vi "ref_gen.vi"(3 "xk":T1, 4 "error in (no error)":errorcluster, 5 "wd":dbl, 6 "B":T1, 7 "A":T1) -> (0 "error out":errorcluster, 1 "xkp1":T1)   [LabVIEW 2021]
uses:
  <vilib>/Analysis/Matrix/Datatypes/RealMatrix.ctl
  <vilib>/Analysis/Matrix/Numeric/Multiply/Multiply - RM,R.vi
  <vilib>/Analysis/Matrix/Numeric/Multiply/Multiply - RM,RM.vi
  <vilib>/Analysis/Matrix/Numeric/Add/Add - RM,RM.vi
  <vilib>/Analysis/Matrix/NI_Matrix.lvlib
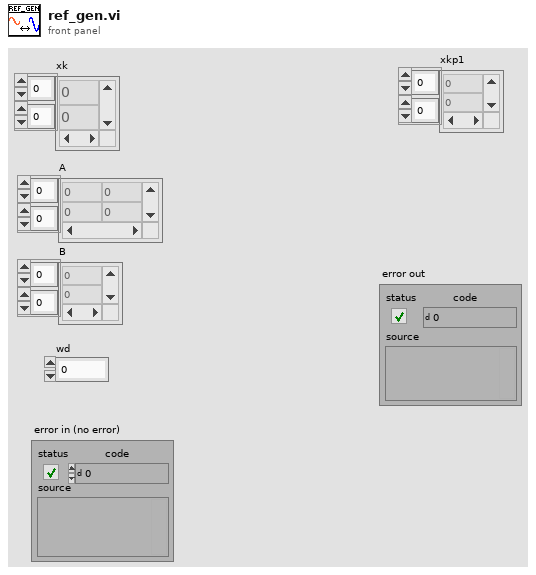
[diagram p1: front panel]
types:
  T1 = typedef "NI_Matrix.lvlib/RealMatrix.ctl" = dbl[][]
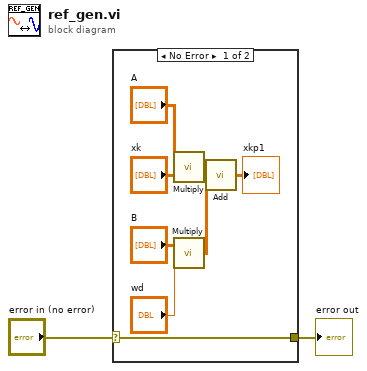
[diagram p0: block diagram]
diagram:
  n1 = case shown="No Error" "error in (no error)" {
    selector: "error in (no error)" -> [w10 w11]
    tunnel: [w10 w11] -> w1
    frame No Error {
      n2 = call-poly <vilib>:"Multiply.vi"("Real Matrix B"="xk", "Real Matrix A"="A") -> ("A * B"=w3:T1)
      n3 = call-poly <vilib>:"Multiply.vi"("Real Scalar c"="wd", "Real Matrix A"="B") -> ("A * c"=w7:T1)
      n4 = call-poly <vilib>:"Add.vi"("Real Matrix B"=w7, "Real Matrix A"=w3) -> ("A + B"=→"xkp1":T1)
    }
    frame Error {
    }
  }
  "error out" <- w1
